vi "Convertir_WResponse_toBool.vi"(10 "Comando Write Response":string, 11 "Valor Actual":bool[](array[boolean])) -> (2 "Canal":i32, 3 "Nuevo Valor":bool[](array[boolean]))   [LabVIEW 2019]
uses:
  <vilib>/regexp/Match Regular Expression.xnode
panel:
  out "Sumar/Restar":bool[](array[boolean])
  out "Estado":bool
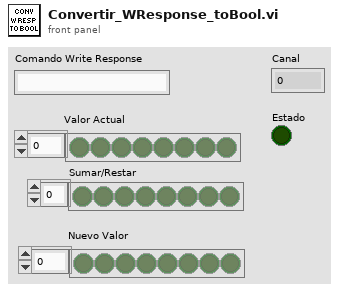
[diagram p1: front panel]
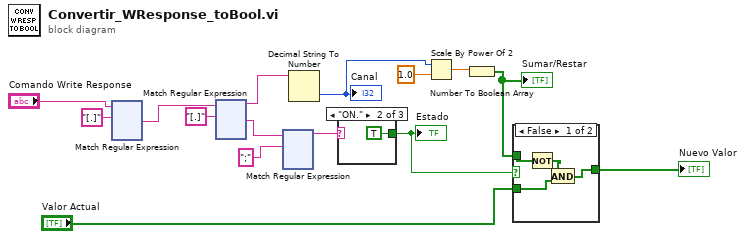
[diagram p0: block diagram]
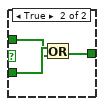
[diagram p2: hidden frame]
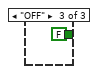
[diagram p4: hidden frame]
diagram:
  n1 = xnode "Match Regular Expression"("input string"="Comando Write Response", "regular expression"="[.]") -> ("after match"=w3:string)  [unwired: 4 in, 4 out]
  n2 = xnode "Match Regular Expression"("input string"=w3, "regular expression"="[.]") -> ("before match"=w5:string, "after match"=w6:string)  [unwired: 4 in, 3 out]
  n3 = xnode "Match Regular Expression"("input string"=w6, "regular expression"=";") -> ("before match"=w8:string)  [unwired: 4 in, 4 out]
  n4 = Decimal String To Number(string=w5) -> (number=w10:i32)  [unwired: 2 in, 1 out]
  "Canal" <- w10
  n5 = case shown="\"ON.\"" w8 {
    tunnel: [_ TRUE FALSE] -> w12
    frame "False", Default {
    }
    frame "ON." {
    }
    frame "OFF" {
    }
  }
  "Estado" <- w12
  n6 = Scale By Power Of 2(n=w10, x=1.0) -> (x*2^n=w11:dbl)
  n7 = Number To Boolean Array(number=w11) -> (Boolean array=w14:bool[])
  "Sumar/Restar" <- w14
  n8 = case shown="False" w12 {
    tunnel: "Valor Actual" -> [w19 w24]
    tunnel: w14 -> [w21 w23]
    tunnel: [w18 w22] -> w15
    frame False {
      n9 = Not(x=w21) -> (.not. x?=w20:bool[])
      n10 = And(x=w20, y=w19) -> (x .and. y?=w18:bool[])
    }
    frame True {
      n11 = Or(x=w24, y=w23) -> (x .or. y?=w22:bool[])
    }
  }
  "Nuevo Valor" <- w15
